vi "MakeSquare.vi"() -> ()   [LabVIEW 2014]
panel:
  in  "milliseconds to wait":u32
  in  "stop":bool
  in  "Amplitude (um)":dbl
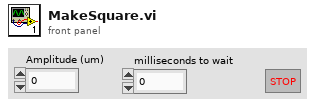
[diagram p1: front panel]
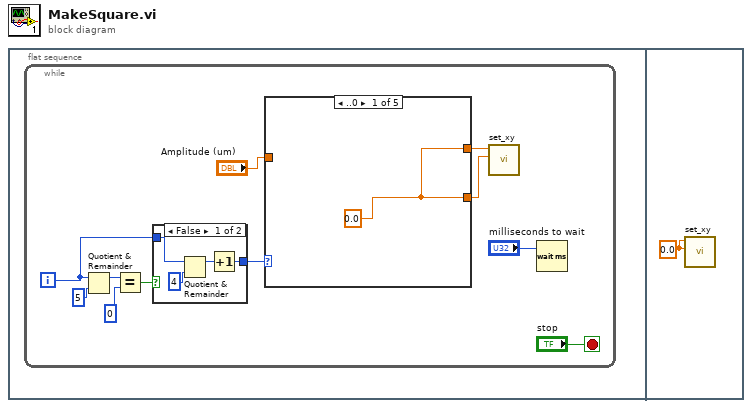
[diagram p0: block diagram]
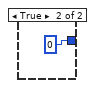
[diagram p2: hidden frame]
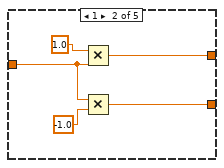
[diagram p3: hidden frame]
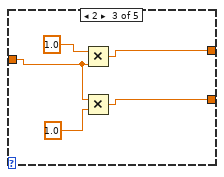
[diagram p4: hidden frame]
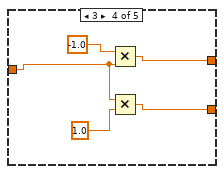
[diagram p5: hidden frame]
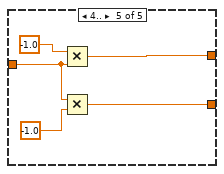
[diagram p6: hidden frame]
diagram:
  n1 = flat-sequence {
    frame #0 {
      n2 = while {
        i -> [w1]
        stop <- "stop" stop-if-true
        n3 = Quotient & Remainder(x=w1, y=5) -> (x-y*floor(x/y)=w2:i32)  [unwired: 1 out]
        n4 = Equal?(x=w2, y=0) -> (x = y?=w4:bool)
        n5 = case shown="False" w4 {
          tunnel: [w12 0 ("y")] -> w3
          tunnel: w1 -> [w14 _]
          frame False {
            n6 = Quotient & Remainder(x=w14, y=4) -> (x-y*floor(x/y)=w15:i32)  [unwired: 1 out]
            n7 = Increment(x=w15) -> (x+1=w12:i32)
          }
          frame True {
          }
        }
        n8 = case shown="..0" w3 {
          tunnel: "Amplitude (um)" -> [_ w20 w25 w30 w33]
          tunnel: [w17 w19 w24 w29 w35] -> w9
          tunnel: [w17 w18 w23 w28 w34] -> w8
          frame ..0 {
            w17 = 0.0
          }
          frame 1 {
            n9 = Multiply(x=1.0 ("y"), y=w20) -> (x*y=w19:dbl)
            n10 = Multiply(x=w20, y=-1.0) -> (x*y=w18:dbl)
          }
          frame 2 {
            n11 = Multiply(x=1.0 ("y"), y=w25) -> (x*y=w24:dbl)
            n12 = Multiply(x=w25, y=1.0) -> (x*y=w23:dbl)
          }
          frame 3 {
            n13 = Multiply(x=-1.0 ("y"), y=w30) -> (x*y=w29:dbl)
            n14 = Multiply(x=w30, y=1.0) -> (x*y=w28:dbl)
          }
          frame 4.. {
            n15 = Multiply(x=-1.0 ("y"), y=w33) -> (x*y=w35:dbl)
            n16 = Multiply(x=w33, y=-1.0) -> (x*y=w34:dbl)
          }
        }
        n17 = call "set_xy.vi"("y_value_um"=w8, "x_value_um"=w9) -> ()  [unwired: 9 in, 1 out]
        n18 = Wait (ms)(milliseconds to wait="milliseconds to wait") -> ()  [unwired: 1 out]
      }
    }
    frame #1 {
      w38 = 0.0
      n19 = call "set_xy.vi"("y_value_um"=w38, "x_value_um"=w38) -> ()  [unwired: 9 in, 1 out]
    }
  }
